vi "PID Advanced Autotuning.vi"(0 "setpoint":dbl, 1 "output range":cluster{"output high":dbl, "output low":dbl}={"output high"=100.0, "output low"=-100.0}, 2 "auto? (F)":bool, 3 "manual control":dbl, 5 "process variable":dbl, 6 "gamma":dbl format="%.2f", 7 "autotune? (F)":bool, 8 "alpha":dbl=0.1 format="%.2f", 9 "PID gains":T2={"proportional gain (Kc)"=1.0, "integral time (Ti, min)"=0.01, "derivative time (Td, min)"=0.0} {"derivative time (Td, min)" format="%#.6g"; "integral time (Ti, min)" format="%#.6g"; "proportional gain (Kc)" format="%#.6g"}, 11 "dt (s)":dbl, 12 "reinitialize? (F)":bool, 13 "beta":dbl=1.0, 14 "autotuning parameters":T1={"technique"=2, "type of controller"=1, "control specification"=0, "amplitude"=1.0} {"amplitude" format="%.2f"; "control specification" items=["normal", "fast", "slow"]; "type of controller" items=["P", "PI", "PID"]; "technique" items=["Step Open Loop", "Step Closed Loop", "Relay", "PID Relay"]}) -> (4 "output":dbl, 10 "tuned PID gains":T2={"proportional gain (Kc)"=1.0, "integral time (Ti, min)"=0.01, "derivative time (Td, min)"=0.0} {"derivative time (Td, min)" format="%#.6g"; "integral time (Ti, min)" format="%#.6g"; "proportional gain (Kc)" format="%#.6g"}, 15 "tuning completed?":bool)   [LabVIEW 2020, in "NI_PID_autopid.lvlib"]
doc: "Implements a PID controller using a PID algorithm with advanced optional features, and applies autotuning to the controller. You can use this VI in RT applications."
uses:
  <vilib>/addons/control/pid/NI_PID_autopid.lvlib
  <vilib>/addons/control/pid/autopid.llb/PID autotuning parameters.ctl
  <vilib>/addons/control/pid/autopid.llb/PID autotuning parameters (adv).ctl
  <vilib>/addons/control/pid/autopid.llb/PID Online Autotuning (Step Open Loop).vi
  <vilib>/addons/control/pid/autopid.llb/PID Online Autotuning (Step Closed Loop).vi
  <vilib>/addons/control/pid/autopid.llb/PID Online Autotuning (Relay Feedback).vi
  <vilib>/addons/control/pid/autopid.llb/PID Online Autotuning (PID on the loop).vi
  <vilib>/addons/control/pid/pid.llb/PID Advanced (DBL).vi
  <vilib>/addons/control/pid/NI_PID_pid.lvlib
  <vilib>/ptbypt/NI_PtbyPt.lvlib
panel:
  in  "autotuning parameters":T3={"type of controller"=1, "relay cycles"=3, "relay amplitude"=1.0, "control specifications"=2, "PV noise level"=0.1} {"PV noise level" format="%.2f"; "control specifications" items=["Fast", "Normal", "Slow"]; "relay amplitude" format="%.2f"; "type of controller" items=["P", "PI", "PID"]}
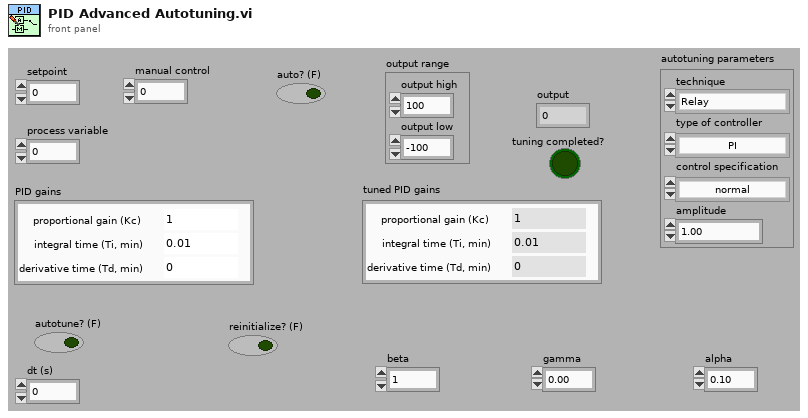
[diagram p1: front panel]
types:
  T1 = typedef "NI_PID_autopid.lvlib/PID autotuning parameters (adv).ctl" = cluster{"technique":u16, "type of controller":u16, "control specification":u16, "amplitude":dbl}
  T2 = cluster{"proportional gain (Kc)":dbl, "integral time (Ti, min)":dbl, "derivative time (Td, min)":dbl}
  T3 = typedef "PID autotuning parameters.ctl" = cluster{"type of controller":u16, "relay cycles":i32, "relay amplitude":dbl, "control specifications":u16, "PV noise level":dbl}
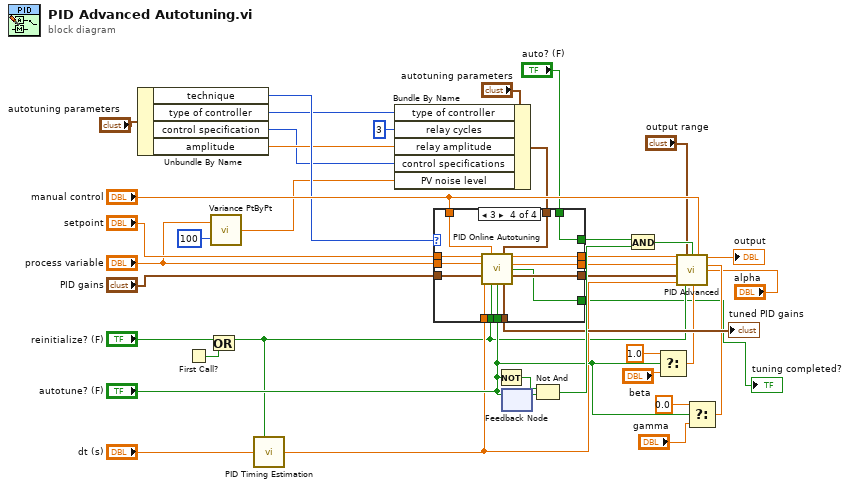
[diagram p0: block diagram]
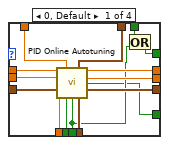
[diagram p2: hidden frame]
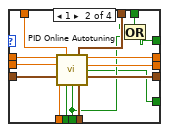
[diagram p3: hidden frame]
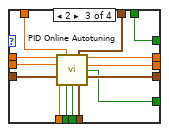
[diagram p4: hidden frame]
diagram:
  n1 = Unbundle By Name("autotuning parameters") -> ("technique"=w20:u16, "type of controller"=w19:u16, "control specification"=w16:u16, "amplitude"=w17:dbl)
  n2 = First Call?() -> (First Call?: T/F=w7:bool)
  n3 = Or(x="reinitialize? (F)", y=w7) -> (x .or. y?=w2:bool)
  n4 = call <vilib>:"Variance PtByPt.vi"("x"="process variable", "sample length"=100) -> ("variance"=w13:dbl)  [unwired: 1 in, 2 out]
  n5 = call <vilib>:"PID Timing Estimation.vi"("Initialize?"=w2, "dt (s) in"="dt (s)") -> ("dt (s) out"=w3:dbl)  [unwired: 7 in]
  n6 = Bundle By Name(cluster="autotuning parameters", "type of controller"=w19, "relay cycles"=3, "relay amplitude"=w17, "control specifications"=w16, "PV noise level"=w13) -> (w22:T3)
  n7 = case shown="3" w20 {
    tunnel: "setpoint" -> [w55 w70 w84 w98]
    tunnel: w3 -> [w54 w69 w83 w97]
    tunnel: "manual control" -> [w53 w68 w82 w96]
    tunnel: "process variable" -> [w52 w67 w81 w95]
    tunnel: [w51 w66 w80 w94] -> w32
    tunnel: [w50 w65 w79 w93] -> w31
    tunnel: "PID gains" -> [w49 w64 w78 w92]
    tunnel: [w48 w63 w77 w91] -> w29
    tunnel: [w47 w62 w76 w90] -> w28
    tunnel: w2 -> [w46 w60 w75 w89]
    tunnel: "autotune? (F)" -> [w44 w57 w74 w88]
    tunnel: w22 -> [w45 w61 w73 w87]
    tunnel: "auto? (F)" -> [w43 w59 w72 w86]
    tunnel: [w42 w58 w72 w86] -> w11
    tunnel: [w41 w56 w71 w85] -> w1
    frame 0, Default {
      n8 = call-poly <vilib>:"PID Online Autotuning.VI"("setpoint"=w55, "manipulated variable"=w53, "autotuning parameters"=w45, "process variable"=w52, "PID gains in"=w49, "dt (s)"=w54, "reinitialize? (F)"=w46, "autotune? (F)"=w44) -> ("setpoint out"=w47:dbl, "process variable out"=w48:dbl, "tuning completed?"=w41:bool, "PID gains out"=w50:T2, "tuned PID gains"=w51:T2)  [unwired: 3 in]
      n9 = Or(x=w43, y=w44) -> (x .or. y?=w42:bool)
    }
    frame 1 {
      n10 = call-poly <vilib>:"PID Online Autotuning.VI"("setpoint"=w70, "manipulated variable"=w68, "autotuning parameters"=w61, "process variable"=w67, "PID gains in"=w64, "dt (s)"=w69, "reinitialize? (F)"=w60, "autotune? (F)"=w57) -> ("setpoint out"=w62:dbl, "process variable out"=w63:dbl, "tuning completed?"=w56:bool, "PID gains out"=w65:T2, "tuned PID gains"=w66:T2)  [unwired: 3 in]
      n11 = Or(x=w59, y=w57) -> (x .or. y?=w58:bool)
    }
    frame 2 {
      n12 = call-poly <vilib>:"PID Online Autotuning.VI"("setpoint"=w84, "manipulated variable"=w82, "autotuning parameters"=w73, "process variable"=w81, "PID gains in"=w78, "dt (s)"=w83, "reinitialize? (F)"=w75, "autotune? (F)"=w74) -> ("setpoint out"=w76:dbl, "process variable out"=w77:dbl, "tuning completed?"=w71:bool, "PID gains out"=w79:T2, "tuned PID gains"=w80:T2)  [unwired: 3 in]
    }
    frame 3 {
      n13 = call-poly <vilib>:"PID Online Autotuning.VI"("setpoint"=w98, "manipulated variable"=w96, "autotuning parameters"=w87, "process variable"=w95, "PID gains in"=w92, "dt (s)"=w97, "reinitialize? (F)"=w89, "autotune? (F)"=w88) -> ("setpoint out"=w90:dbl, "process variable out"=w91:dbl, "tuning completed?"=w85:bool, "PID gains out"=w93:T2, "tuned PID gains"=w94:T2)  [unwired: 3 in]
    }
  }
  "tuned PID gains" <- w32
  "tuning completed?" <- w1
  n14 = Not(x="autotune? (F)") -> (.not. x?=w39:bool)
  n15 = feedback #1() -> (w37:bool)  [unwired: 1 in]
  n16 = feedback-in #1("autotune? (F)") -> ()
  n17 = Not And(1:w37, 2:w39) -> (0:w38:bool)
  n18 = And(x=w11, y=w38) -> (x .and. y?=w36:bool)
  n19 = Select(t=1.0, s="autotune? (F)", f="beta") -> (s? t:f=w24:dbl)
  n20 = Select(t=0.0, s="autotune? (F)", f="gamma") -> (s? t:f=w6:dbl)
  n21 = call-poly <vilib>:"PID Advanced.vi"("setpoint"=w28, "output range"="output range", "auto? (T)"=w36, "manual control"="manual control", "process variable"=w29, "gamma"=w6, "alpha"="alpha", "PID gains"=w31, "dt (s)"=w3, "reinitialize? (F)"=w2, "beta"=w24) -> ("output"=→"output":dbl)  [unwired: 3 in, 1 out]
